vi "Read Use Tiered Panels_.vi"(8 "error in (no error)":errorcluster, 11 "Panel Form Controller Configuration in":refnum<class "Panel Form Controller Configuration.lvclass">) -> (0 "error out":errorcluster, 2 "Use Tiered Panels?":bool, 3 "Panel Form Controller Configuration out":refnum<class "Panel Form Controller Configuration.lvclass">)   [LabVIEW 2020, in "Panel Form Controller.lvlib" / "Panel Form Controller Configuration.lvclass"]
uses:
  Panel Form Controller Configuration.lvclass
  Panel Form Controller Configuration.lvclass/Panel Form Controller Configuration.ctl
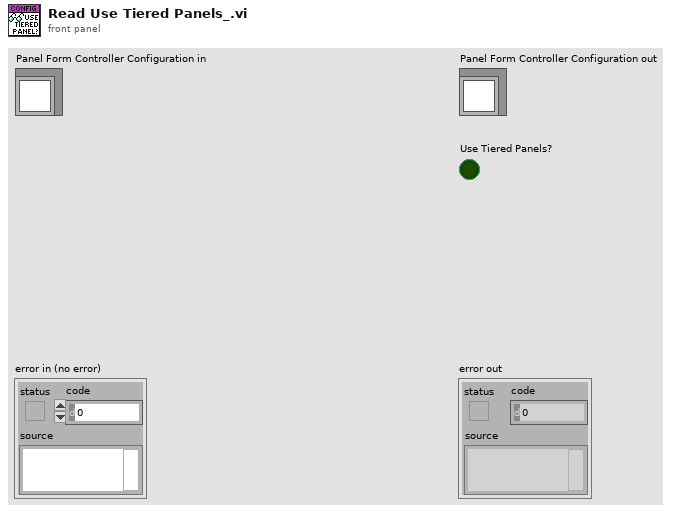
[diagram p1: front panel]
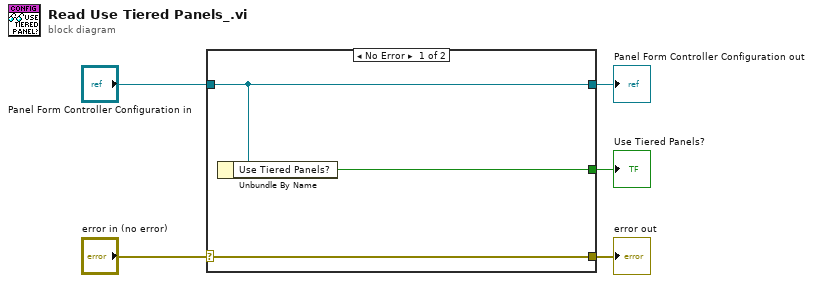
[diagram p0: block diagram]
diagram:
  n1 = case shown="No Error" "error in (no error)" {
    selector: "error in (no error)" -> [w8 w9]
    tunnel: [w8 w9] -> w4
    tunnel: [w7 w10] -> w2
    tunnel: "Panel Form Controller Configuration in" -> [w7 w10]
    tunnel: [w6 _] -> w1
    frame No Error {
      n2 = Unbundle By Name(w7) -> ("Use Tiered Panels?"=w6:bool)
    }
    frame Error {
    }
  }
  "error out" <- w4
  "Panel Form Controller Configuration out" <- w2
  "Use Tiered Panels?" <- w1
